vi "Pr Data Global.vi"() -> ()   [LabVIEW 2013]
panel:
  out "Reset":bool[](array[boolean])
  in  "Data 10":sgl[](array[numeric])=[0.0, 0.0, 0.0] format="%.2f"
  in  "Data 9":sgl[](array[numeric])=[0.0, 0.0, 0.0] format="%.2f"
  in  "Data 8":sgl[](array[numeric])=[0.0, 0.0, 0.0] format="%.2f"
  in  "Data 7":sgl[](array[numeric])=[0.0, 0.0, 0.0] format="%.2f"
  in  "Data 6":sgl[](array[numeric])=[0.0, 0.0, 0.0] format="%.2f"
  in  "Data 5":sgl[](array[numeric])=[0.0, 0.0, 0.0] format="%.2f"
  in  "Data 4":sgl[](array[numeric])=[0.0, 0.0, 0.0] format="%.2f"
  in  "Data 3":sgl[](array[numeric])=[0.0, 0.0, 0.0] format="%.2f"
  in  "Data 2":sgl[](array[numeric])=[0.0, 0.0, 0.0] format="%.2f"
  in  "Data 1":sgl[](array[numeric])=[0.0, 0.0, 0.0] format="%.2f"
  # "max."
  # "ave."
  # "min."
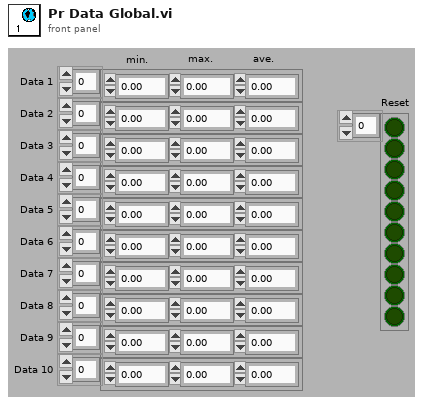
[diagram p1: front panel]
diagram:
